vi "Find Goals.vi"(6 "Aspect Fudge Factor":dbl=1.0, 8 "Score Threshold":dbl=75.0 format="%#_13g", 9 "Color":T3, 10 "Image Dst":T2, 11 "Image Src":T2) -> (2 "Targets":T1(array[cluster]), 3 "Masked Image":T2)   [LabVIEW 2015]
uses:
  <vilib>/vision/Image Controls.llb/IMAQ Image.ctl
  <vilib>/vision/NI_Vision_Development_Module.lvlib
panel:
  out "error out":errorcluster
  out "Particles":i32
  out "Highest Avg":dbl
  in  "Emphasize Limit Tests":bool=TRUE
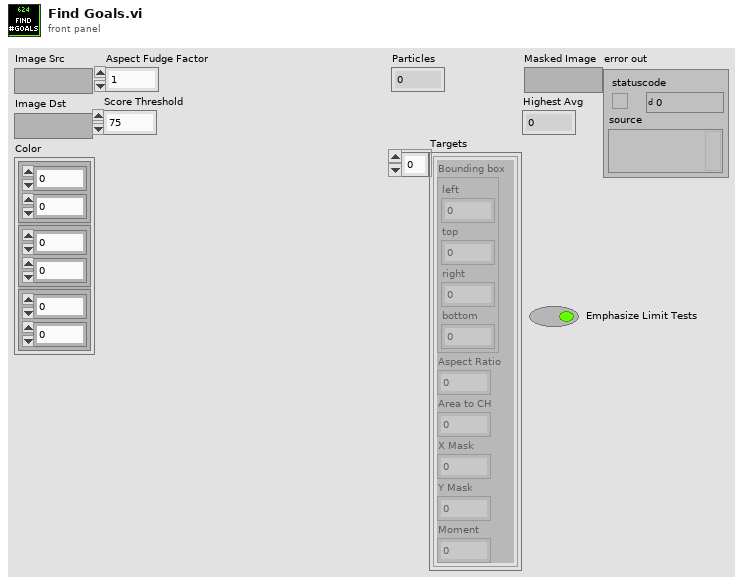
[diagram p1: front panel]
types:
  T1 = cluster{"Bounding box":cluster{"left":dbl, "top":dbl, "right":dbl, "bottom":dbl}, "Aspect Ratio":dbl, "Area to CH":dbl, "X Mask":dbl, "Y Mask":dbl, "Moment":dbl}[]
  T2 = typedef "IMAQ Image.ctl" = refnum<image>
  T3 = cluster{cluster{dbl, dbl}, cluster{dbl, dbl}, cluster{dbl, dbl}}
  T4 = typedef "Particle Parameters" = i32
  T5 = cluster{"left":dbl, "top":dbl, "right":dbl, "bottom":dbl}
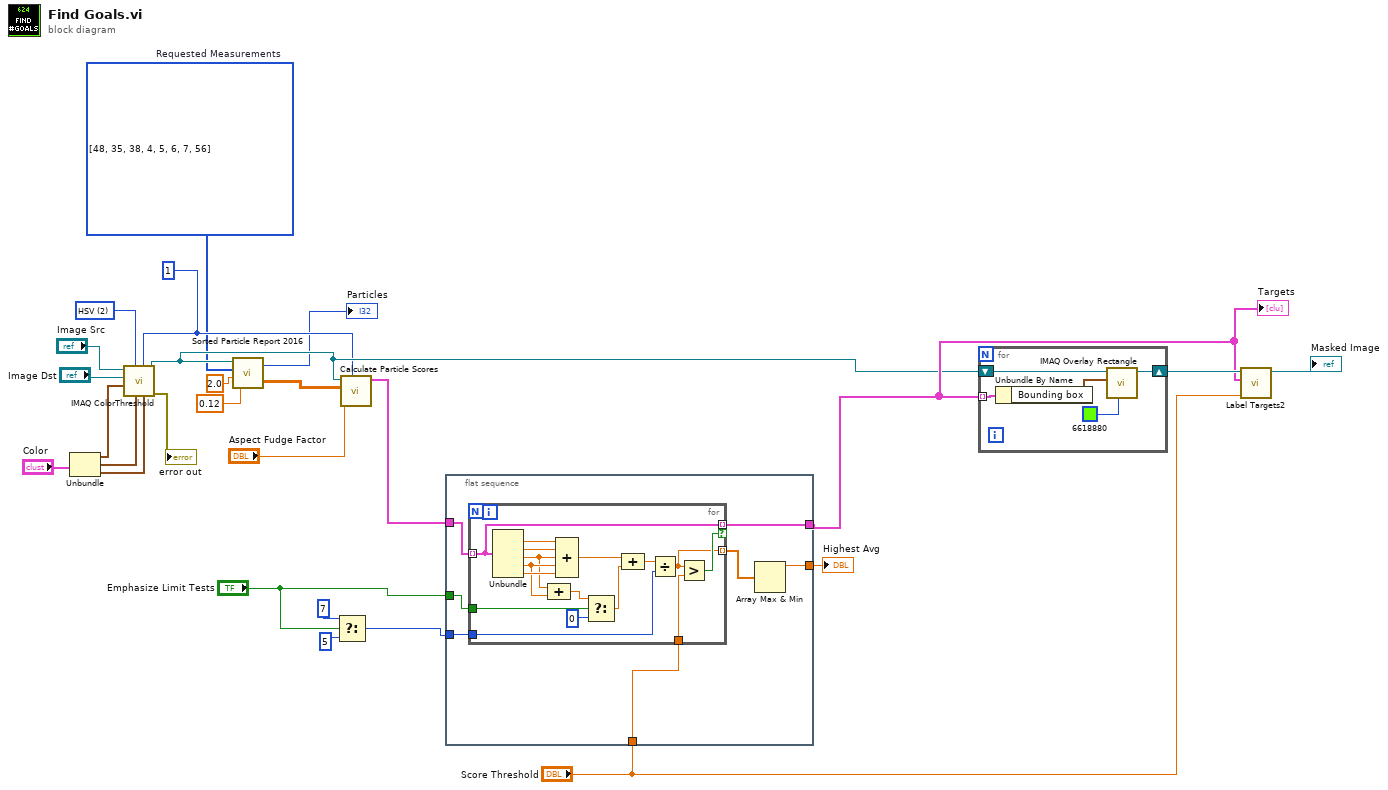
[diagram p0: block diagram]
diagram:
  w2 = T4[] [48, 35, 38, 4, 5, 6, 7, 56] items=["Center of Mass X", "Center of Mass Y", "First Pixel X", "First Pixel Y", "Bounding Rect Left", "Bounding Rect Top", "Bounding Rect Right", "Bounding Rect Bottom", "Max Feret Diameter Start X", "Max Feret Diameter Start Y", "Max Feret Diameter End X", "Max Feret Diameter End Y", "Max Horiz. Segment Length Left", "Max Horiz. Segment Length Right", "Max Horiz. Segment Length Row", "-", "Bounding Rect Width", "Bounding Rect Height", "Bounding Rect Diagonal", "Perimeter", "Convex Hull Perimeter", "Holes' Perimeter", "Max Feret Diameter", "Equivalent Ellipse Major Axis", "Equivalent Ellipse Minor Axis", "Equivalent Ellipse Minor Axis (Feret)", "Equivalent Rect Long Side", "Equivalent Rect Short Side", "Equivalent Rect Diagonal", "Equivalent Rect Short Side (Feret)", "Average Horiz. Segment Length", "Average Vert. Segment Length", "Hydraulic Radius", "Waddel Disk Diameter", "-", "Area", "Holes' Area", "Particle & Holes' Area", "Convex Hull Area", "Image Area", "-", "Number of Holes", "Number of Horiz. Segments", "Number of Vert. Segments", "-", "Orientation", "Max Feret Diameter Orientation", "-", "% Area/Image Area", "% Area/(Particle & Holes' Area)", "Ratio of Equivalent Ellipse Axes", "Ratio of Equivalent Rect Sides", "-", "Elongation Factor", "Compactness Factor", "Heywood Circularity Factor", "Type Factor", "-", "Sum X", "Sum Y", "Sum XX", "Sum XY", "Sum YY", "Sum XXX", "Sum XXY", "Sum XYY", "Sum YYY", "-", "Moment of Inertia XX", "Moment of Inertia XY", "Moment of Inertia YY", "Moment of Inertia XXX", "Moment of Inertia XXY", "Moment of Inertia XYY", "Moment of Inertia YYY", "Norm. Moment of Inertia XX", "Norm. Moment of Inertia XY", "Norm. Moment of Inertia YY", "Norm. Moment of Inertia XXX", "Norm. Moment of Inertia XXY", "Norm. Moment of Inertia XYY", "Norm. Moment of Inertia YYY", "Hu Moment 1", "Hu Moment 2", "Hu Moment 3", "Hu Moment 4", "Hu Moment 5", "Hu Moment 6", "Hu Moment 7"]  # Requested Measurements
  w4 = 1 ("Pixel Value")
  w24 = u16 2 items=["RGB", "HSL", "HSV", "HSI"] ("Color Mode")
  n1 = Unbundle("Color") -> (w22:cluster{dbl, dbl}, w21:cluster{dbl, dbl}, w20:cluster{dbl, dbl})
  n2 = call "IMAQ ColorThreshold"("Blue or Luma or Val or Inten Range"=w20, "Replace Value"=w4, "Green or Sat Range"=w21, "Color Mode"=w24, "Red or Hue Range"=w22, "Image Dst"="Image Dst", "Image Src"="Image Src") -> ("error out"=→"error out":errorcluster, "Image Dst Out"=w6:T2)  [unwired: 3 in]
  n3 = call "Sorted Particle Report 2016.vi"("Min Area Size %"=0.12, "Particle Count Limit"=2.0, "Pixel Measurements"=w2, "Image in"=w6) -> ("Sorted Data"=w17:dbl[][], "Particles"=→"Particles":i32)
  n4 = Select(t=7, s="Emphasize Limit Tests", f=5) -> (s? t:f=w12:i32)
  n5 = call "Calculate Particle Scores.vi"("Pixel Value"=w4, "Aspect Fudge Factor"="Aspect Fudge Factor", "Sorted Data"=w17, "Image in"=w6) -> ("Scores"=w5:T1)  [unwired: 7 in]
  n6 = flat-sequence {
    tunnel: w5 -> [w32]
    tunnel: w12 -> [w30]
    tunnel: [w33] -> w11
    tunnel: [w28] -> w7
    tunnel: "Emphasize Limit Tests" -> [w31]
    tunnel: "Score Threshold" -> [w27]
    frame #0 {
      n7 = for {
        tunnel: w32 -> [w47] mode=indexing
        tunnel: [w47] -> w28 mode=indexing if=w46
        tunnel: [w45] -> w29 mode=indexing
        tunnel: w30 -> [w44]
        tunnel: w27 -> [w43]
        tunnel: w31 -> [w36]
        n8 = Unbundle(w47) -> ("Aspect Ratio"=w49:dbl, "Area to CH"=w48:dbl, "X Mask"=w38:dbl, "Y Mask"=w39:dbl, "Moment"=w40:dbl)  [unwired: 1 out]
        n9 = Compound Arithmetic op=ADD(w38, w39) -> (w37:dbl)
        n10 = Compound Arithmetic op=ADD(w49, w48, w38, w39, w40) -> (w42:dbl)
        n11 = Select(t=w37, s=w36, f=0) -> (s? t:f=w35:dbl)
        n12 = Compound Arithmetic op=ADD(w42, w35) -> (w41:dbl)
        n13 = Divide(x=w41, y=w44) -> (x/y=w45:dbl)
        n14 = Greater?(x=w45, y=w43) -> (0:w46:bool)
      }
      n15 = Array Max & Min(array=w29) -> (max value=w33:dbl)  [unwired: 3 out]
    }
  }
  n16 = for {
    shift-right: [w53] -> w10
    shift-left: w6 -> [w54]
    tunnel: w7 -> [w50] mode=indexing
    n17 = Unbundle By Name(w50) -> ("Bounding box"=w52:T5)
    n18 = call "IMAQ Overlay Rectangle"("Color"=u32 6618880, "Rectangle"=w52, "Image"=w54) -> ("Image Out"=w53:T2)  [unwired: 7 in, 1 out]
  }
  n19 = call "Label Targets2.vi"("Score Threshold"="Score Threshold", "Targets"=w7, "Image in"=w10) -> ("Image out"=→"Masked Image":T2)  [unwired: 8 in]
  "Highest Avg" <- w11
  "Targets" <- w7
